vi "Set Driver VIs Dependent File Paths - 331.vi"(8 "error in (no error)":errorcluster, 11 "Item Ref in":T1 format="%.0x") -> (0 "error out":errorcluster, 3 "Item Ref out":T1 format="%.0x")   [LabVIEW 2018, in "FPGA Addon Shared.lvlib"]
uses:
  FPGA Addon Shared.lvlib
  <vilib>/NI Veristand/Custom Device API/Custom Device Item Ref.ctl
  <vilib>/NI Veristand/Custom Device API/Custom Device API.lvlib
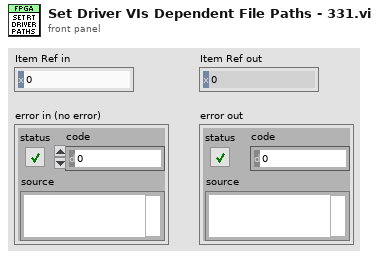
[diagram p1: front panel]
types:
  T1 = typedef "Custom Device API.lvlib/Custom Device Item Ref.ctl" = u64
  T2 = typedef "Advanced System Definition.lvlib/Property.DependentFile.ctl" = cluster{"Original Path":path, "Version":string, "RTDestination":path, "ForceDownload":bool, "SupportedTarget":string, "MD5":string}
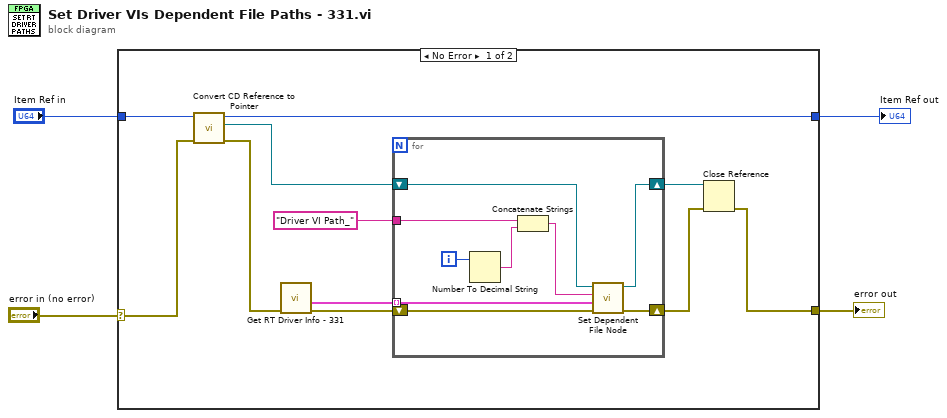
[diagram p0: block diagram]
diagram:
  n1 = case shown="No Error" "error in (no error)" {
    selector: "error in (no error)" -> [w5 w25]
    tunnel: [w14 w25] -> w4
    tunnel: [w11 w26] -> w3
    tunnel: "Item Ref in" -> [w9 w26]
    frame No Error {
      n2 = call "Convert CD Reference to Pointer.vi"("error in (no error)"=w5, "Item Ref in"=w9) -> ("error out"=w12:errorcluster, ".NET Refnum out"=w10:refnum<k24>, "Item Ref out"=w11:T1)  [unwired: 7 in]
      n3 = call "Get RT Driver Info - 331.vi"("error in (no error)"=w12) -> ("error out"=w6:errorcluster, "RT Driver Info"=w7:T2[])  [unwired: 9 in]
      n4 = for {
        shift-right: [w23] -> w13
        shift-left: w6 -> [w24]
        tunnel: w7 -> [w21] mode=indexing
        tunnel: "Driver VI Path_" ("Property name") -> [w20]
        shift-right: [w17] -> w15
        shift-left: w10 -> [w22]
        i -> [w16]
        n5 = Number To Decimal String(number=w16) -> (decimal integer string=w19:string)  [unwired: 1 in]
        n6 = Concatenate Strings(w20, w19) -> (w18:string)
        n7 = call "Set Dependent File Node.vi"("error in (no error)"=w24, "Dependent File info"=w21, "Property name"=w18, ".NET Refnum in"=w22) -> ("error out"=w23:errorcluster, ".NET Refnum out"=w17:refnum<k24>)  [unwired: 5 in, 1 out]
      }
      n8 = Close Reference(reference=w15, error in (no error)=w13) -> (error out=w14:errorcluster)
    }
    frame Error {
    }
  }
  "error out" <- w4
  "Item Ref out" <- w3
